vi "Create Message-Enqueuer References.vi"(8 "error in (no error)":errorcluster) -> (0 "error out":errorcluster, 2 "Messages":T1, 3 "API":T2)   [LabVIEW 2018, in "Scripting.lvlib" / "Actor.lvclass"]
uses:
  Actor.lvclass
  Message-Enqueuer References.ctl
  Stop.ctl
  Launch.ctl
  Did Initialize.ctl
  Messages.ctl
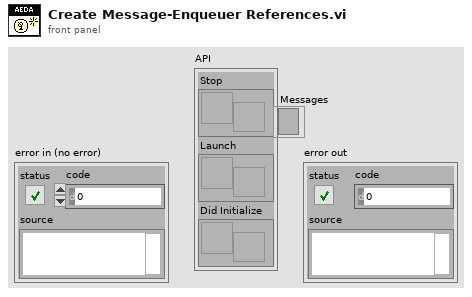
[diagram p1: front panel]
types:
  T1 = typedef "Scripting.lvlib/Actor.lvclass/Messages.ctl" = refnum<event-registration>
  T2 = typedef "Scripting.lvlib/Actor.lvclass/Message-Enqueuer References.ctl" = cluster{"Stop":refnum<user-event>, "Launch":refnum<user-event>, "Did Initialize":refnum<user-event>}
  T3 = typedef "Scripting.lvlib/Actor.lvclass/Launch.ctl" = cluster{"Caller":refnum<vi>}
  T4 = typedef "Scripting.lvlib/Actor.lvclass/Did Initialize.ctl" = cluster{"State":refnum<class "Actor.lvclass">}
  T5 = typedef "Scripting.lvlib/Actor.lvclass/Stop.ctl" = cluster{"Type":enum16{"Normal", "Emergency"}}
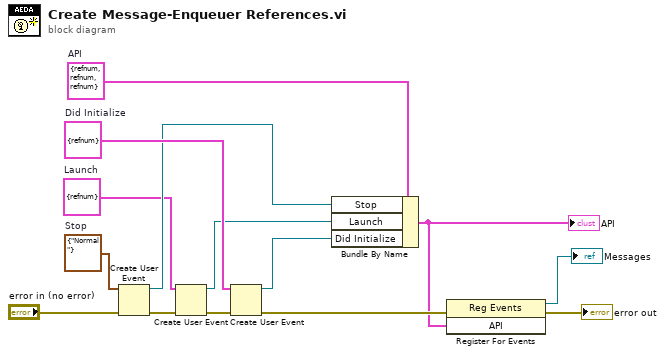
[diagram p0: block diagram]
diagram:
  w5 = T3 {"Caller"=refnum}  # Launch
  w14 = T4 {"State"=refnum}  # Did Initialize
  w13 = T5 {"Type"=enum."Normal"}  # Stop
  w11 = T2 {"Stop"=refnum, "Launch"=refnum, "Did Initialize"=refnum}  # API
  n1 = Create User Event(user event datatype=w13, error in="error in (no error)") -> (user event=w10:refnum<user-event>, error out=w8:errorcluster)
  n2 = Create User Event(user event datatype=w5, error in=w8) -> (user event=w6:refnum<user-event>, error out=w7:errorcluster)
  n3 = Create User Event(user event datatype=w14, error in=w7) -> (user event=w9:refnum<user-event>, error out=w4:errorcluster)
  n4 = Bundle By Name(cluster=w11, "Stop"=w10, "Launch"=w6, "Did Initialize"=w9) -> (w2:T2)
  "API" <- w2
  n5 = register-events(error in=w4, w2) -> (reference out=→"Messages":refnum<event-registration>, error out=→"error out":errorcluster)  [unwired: 1 in]
